vi "Configure Temperature Units.vi"(0 "VISA resource name":refnum<visa-resource-name>, 1 "Units (0:Celsius)":enum16{"Celsius", "Fahrenheit", "Kelvin"}(ring)=enum."Fahrenheit", 2 "Channel List(empty) in":string, 3 "error in (no error)":errorcluster) -> (5 "VISA resource name out":refnum<visa-resource-name>, 8 "error out":errorcluster)   [LabVIEW 2016, in "Agilent 34970.lvlib"]
uses:
  Agilent 34970.lvlib
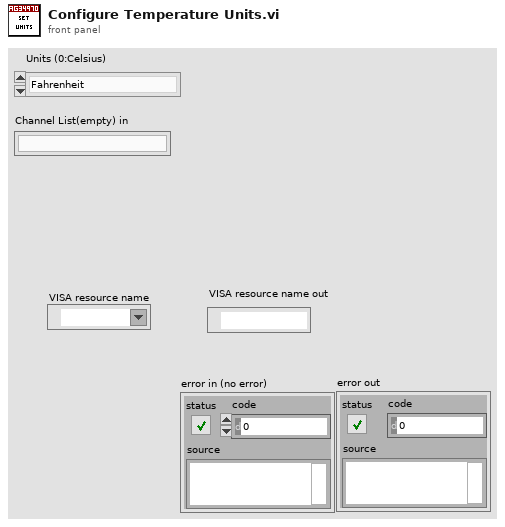
[diagram p1: front panel]
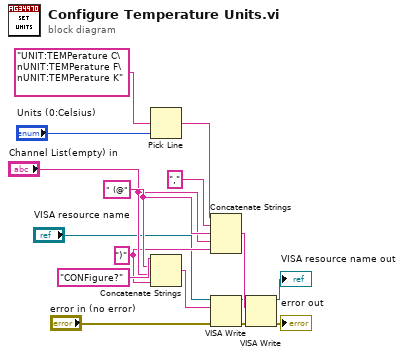
[diagram p0: block diagram]
diagram:
  w6 = ")"
  w8 = " (@"
  n1 = Pick Line(multi-line string="UNIT:TEMPerature C\nUNIT:TEMPerature F\nUNIT:TEMPerature K", line index="Units (0:Celsius)") -> (output string=w14:string)  [unwired: 1 in]
  n2 = Concatenate Strings("CONFigure?" ("string"), w8, "Channel List(empty) in", w6) -> (w3:string)
  n3 = Concatenate Strings(w14, "," ("string"), w8, "Channel List(empty) in", w6) -> (w13:string)
  n4 = VISA Write(VISA resource name="VISA resource name", write buffer=w3, error in (no error)="error in (no error)") -> (VISA resource name out=w4:refnum<visa-resource-name>, error out=w1:errorcluster)  [unwired: 1 out]
  n5 = VISA Write(VISA resource name=w4, write buffer=w13, error in (no error)=w1) -> (VISA resource name out=→"VISA resource name out":refnum<visa-resource-name>, error out=→"error out":errorcluster)  [unwired: 1 out]
